vi "snap.vi"(7 "N":i32, 8 "error in (no error)":errorcluster, 10 "Buffer":u16[][](array[numeric]), 11 "Handle in":u32) -> (0 "error out":errorcluster, 2 "data":dbl[][](array[numeric]))   [LabVIEW 2012]
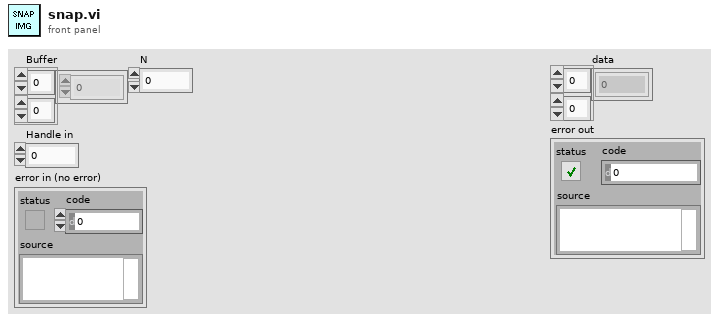
[diagram p1: front panel]
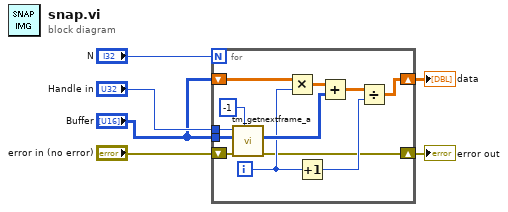
[diagram p0: block diagram]
diagram:
  n1 = for {
    N: "N" -> [_]
    tunnel: "Buffer" -> [w18]
    tunnel: "Handle in" -> [w17]
    shift-right: [w9] -> w2
    shift-left: "Buffer" -> [w15]
    shift-right: [w8] -> w1
    shift-left: "error in (no error)" -> [w16]
    i -> [w11]
    n2 = call "tm_getnextframe_a.vi"("Timeout"=-1, "error in (no error)"=w16, "Buffer"=w18, "Handle in"=w17) -> ("error out"=w8:errorcluster, "Data"=w13:u16[][])  [unwired: 5 in, 1 out]
    n3 = Multiply(x=w15, y=w11) -> (x*y=w14:dbl[][])
    n4 = Increment(x=w11) -> (x+1=w10:i32)
    n5 = Add(x=w14, y=w13) -> (x+y=w12:dbl[][])
    n6 = Divide(x=w12, y=w10) -> (x/y=w9:dbl[][])
  }
  "data" <- w2
  "error out" <- w1
